vi "LV TCP Server.vi"() -> ()   [LabVIEW 2014]
panel:
  out "Data Received":string[](array[string])
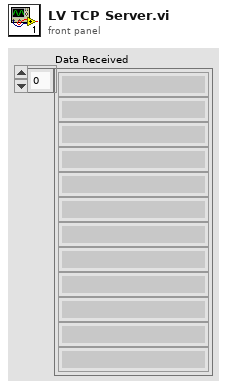
[diagram p1: front panel]
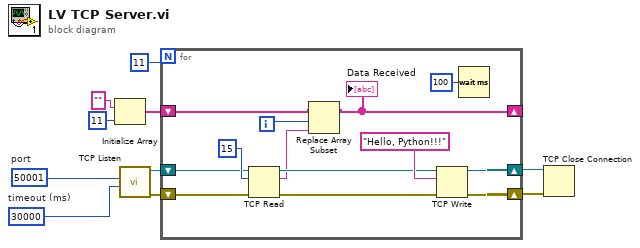
[diagram p0: block diagram]
diagram:
  w9 = u16 50001  # port
  w10 = 30000  # timeout (ms)
  n1 = Initialize Array "Initialize Array"("", 11 ("dimension size")) -> (w3:string[])
  n2 = call <vilib>:"TCP Listen.vi"("timeout ms (wait forever: -1)"=w10, "port"=w9) -> ("error out"=w7:errorcluster, "connection ID"=w8:refnum<k5>)  [unwired: 5 in, 3 out]
  n3 = for {
    N: 11 -> [_]
    shift-right: [w16] -> w6
    shift-left: w8 -> [w21]
    shift-right: [w15] -> w5
    shift-left: w7 -> [w20]
    shift-right: [w13] -> _
    shift-left: w3 -> [w14]
    i -> [w11]
    n4 = TCP Read(connection ID=w21, bytes to read=15, error in (no error)=w20) -> (connection ID out=w18:refnum<k5>, data out=w12:string, error out=w17:errorcluster)  [unwired: 2 out]
    n5 = Replace Array Subset "Replace Array Subset"(array=w14, new element=w12, index=w11) -> (w13:string[])
    "Data Received" <- w13
    n6 = TCP Write(connection ID=w18, data in="Hello, Python!!!", error in (no error)=w17) -> (connection ID out=w16:refnum<k5>, error out=w15:errorcluster)  [unwired: 2 out]
    n7 = Wait (ms)(milliseconds to wait=u32 100) -> ()  [unwired: 1 out]
  }
  n8 = TCP Close Connection(connection ID=w6, error in (no error)=w5) -> ()  [unwired: 3 out]
